vi "BCtr_Disable.vi"(8 "error in (no error)":errorcluster, 11 "CtrCfg":T1 {"BaseAddrOut" format="%x"}) -> (0 "error out":errorcluster, 3 "Ack":bool)   [LabVIEW 2016]
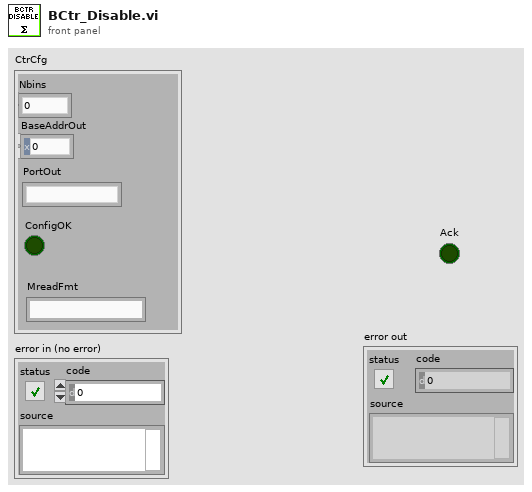
[diagram p1: front panel]
types:
  T1 = cluster{"Nbins":u16, "BaseAddrOut":u16, "PortOut":string, "ConfigOK":bool, "MreadFmt":string}
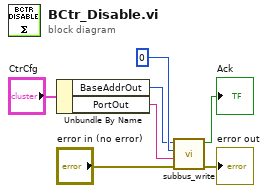
[diagram p0: block diagram]
diagram:
  n1 = Unbundle By Name("CtrCfg") -> ("BaseAddrOut"=w4:u16, "PortOut"=w6:string)
  n2 = call "subbus_write.vi"("error in (no error)"="error in (no error)", "PortIn"=w6, "Data"=0, "Address"=w4) -> ("error out"=→"error out":errorcluster, "Ack"=→"Ack":bool)  [unwired: 5 in, 1 out]
